vi "Register gRPC Methods.vi"(8 "error in (no error)":errorcluster, 11 "Template Server in":refnum<class "Launcher.lvclass">) -> (0 "error out":errorcluster, 3 "Template Server out":refnum<class "Launcher.lvclass">)   [LabVIEW 2021, in "CIF_Launcher_server.lvlib" / "Launcher.lvclass"]
uses:
  Launcher.lvclass
  typeDefs/Server Internal UEs.ctl
  typeDefs/Server Internal Message.ctl
  typeDefs/Server gRPC UEs.ctl
  <vilib>/gRPC/LabVIEW gRPC Library/Server API/typeDefs/gRPCId Cluster.ctl
  <vilib>/gRPC/LabVIEW gRPC Library/Shared/grpcId.ctl
  Launcher.lvclass/Launcher.ctl
  <vilib>/gRPC/LabVIEW gRPC Library/grpc-lvsupport-release.lvlib
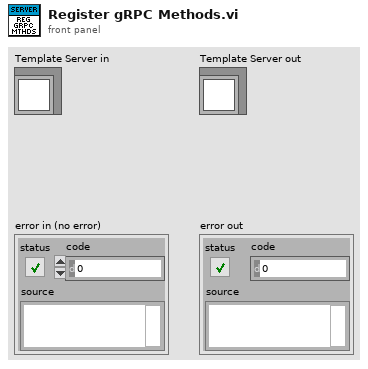
[diagram p1: front panel]
types:
  T1 = typedef "CIF_Launcher_server.lvlib/Launcher.lvclass/Server gRPC UEs.ctl" = cluster{"Launcher LaunchPlugin gRPC UE":refnum<user-event>, "Launcher AbortPlugin gRPC UE":refnum<user-event>, "Launcher Destroy gRPC UE":refnum<user-event>, "Launcher Ping gRPC UE":refnum<user-event>, "Launcher Discover gRPC UE":refnum<user-event>}
  T2 = typedef "CIF_Launcher_server.lvlib/Launcher.lvclass/Server Internal UEs.ctl" = cluster{"Launcher LaunchPlugin Internal UE":refnum<user-event>, "Launcher AbortPlugin Internal UE":refnum<user-event>, "Launcher Destroy Internal UE":refnum<user-event>, "Launcher Ping Internal UE":refnum<user-event>, "Launcher Discover Internal UE":refnum<user-event>}
  T3 = typedef "grpc-lvsupport-release.lvlib/grpcId.ctl" = u64
  T4 = typedef "CIF_Launcher_server.lvlib/Launcher.lvclass/Server Internal Message UE.ctl" = refnum<user-event>
  T5 = typedef "grpc-lvsupport-release.lvlib/gRPCId Cluster UE.ctl" = refnum<user-event>
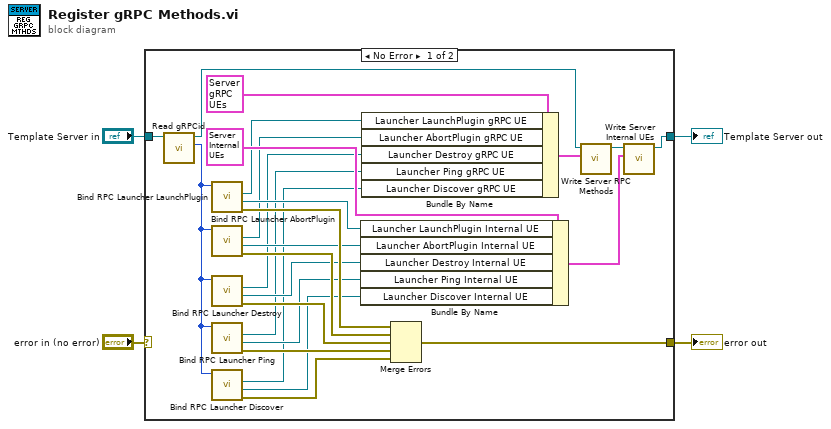
[diagram p0: block diagram]
diagram:
  n1 = case shown="No Error" "error in (no error)" {
    selector: "error in (no error)" -> [_ w30]
    tunnel: "Template Server in" -> [w21 w31]
    tunnel: [w29 w30] -> w3
    tunnel: [w28 w31] -> w2
    frame No Error {
      n2 = call-dynamic "Read gRPCid.vi"("iService in"=w21) -> ("gRPCid"=w20:T3, "iService out"=w22:refnum<class "Launcher.lvclass">)  [unwired: 8 in, 1 out]
      n3 = call "Bind RPC Launcher LaunchPlugin.vi"("gRPCid server in"=w20) -> ("error out"=w19:errorcluster, "Launcher LaunchPlugin Internal UE"=w17:T4, "Launcher LaunchPlugin gRPC UE"=w18:T5)  [unwired: 7 in, 1 out]
      n4 = call "Bind RPC Launcher AbortPlugin.vi"("gRPCid server in"=w20) -> ("error out"=w16:errorcluster, "Launcher AbortPlugin Internal UE"=w14:T4, "Launcher AbortPlugin gRPC UE"=w15:T5)  [unwired: 7 in, 1 out]
      n5 = call "Bind RPC Launcher Destroy.vi"("gRPCid server in"=w20) -> ("error out"=w13:errorcluster, "Launcher Destroy Internal UE"=w11:T4, "Launcher Destroy gRPC UE"=w12:T5)  [unwired: 7 in, 1 out]
      n6 = call "Bind RPC Launcher Ping.vi"("gRPCid server in"=w20) -> ("error out"=w10:errorcluster, "Launcher Ping Internal UE"=w8:T4, "Launcher Ping gRPC UE"=w9:T5)  [unwired: 7 in, 1 out]
      n7 = call "Bind RPC Launcher Discover.vi"("gRPCid server in"=w20) -> ("error out"=w7:errorcluster, "Launcher Discover Internal UE"=w5:T4, "Launcher Discover gRPC UE"=w6:T5)  [unwired: 7 in, 1 out]
      n8 = Bundle By Name ("Bundle Internal UEs")(cluster=T2 {"Launcher LaunchPlugin Internal UE"=refnum, "Launcher AbortPlugin Internal UE"=refnum, "Launcher Destroy Internal UE"=refnum, "Launcher Ping Internal UE"=refnum, "Launcher Discover Internal UE"=refnum} ("Server Internal UEs"), "Launcher LaunchPlugin Internal UE"=w17, "Launcher AbortPlugin Internal UE"=w14, "Launcher Destroy Internal UE"=w11, "Launcher Ping Internal UE"=w8, "Launcher Discover Internal UE"=w5) -> (w27:T2)
      n9 = Bundle By Name ("Bundle gRPC UEs")(cluster=T1 {"Launcher LaunchPlugin gRPC UE"=refnum, "Launcher AbortPlugin gRPC UE"=refnum, "Launcher Destroy gRPC UE"=refnum, "Launcher Ping gRPC UE"=refnum, "Launcher Discover gRPC UE"=refnum} ("gRPC Server Method Events"), "Launcher LaunchPlugin gRPC UE"=w18, "Launcher AbortPlugin gRPC UE"=w15, "Launcher Destroy gRPC UE"=w12, "Launcher Ping gRPC UE"=w9, "Launcher Discover gRPC UE"=w6) -> (w24:T1)
      n10 = Merge Errors(w19, w16, w13, w10, w7) -> (w29:errorcluster)
      n11 = call "Write Server RPC Methods.vi"("Server RPC Methods"=w24, "SignalGeneratorService in"=w22) -> ("SignalGeneratorService out"=w25:refnum<class "Launcher.lvclass">)  [unwired: 8 in, 1 out]
      n12 = call "Write Server Internal UEs.vi"("Server Internal UEs"=w27, "SignalGeneratorService in"=w25) -> ("SignalGeneratorService out"=w28:refnum<class "Launcher.lvclass">)  [unwired: 8 in, 1 out]
    }
    frame Error {
    }
  }
  "error out" <- w3
  "Template Server out" <- w2
